vi "autodetector.vi"() -> ()   [LabVIEW 2013]
uses:
  TDMS datalogger/module/configuration/TDMS datalogger configuration.lvclass
  TDMS datalogger/module/execution/TDMS datalogger runtime.lvclass
  configuration/Scan Engine configuration.lvclass
  execution/Scan Engine runtime.lvclass
  <vilib>/NI/Tag Bus Module Framework/channel/TBM channel.lvclass
  <vilib>/NI/Tag Bus/tag/Data Type.ctl
  <vilib>/NI/Tag Bus/tag/tag descriptor.lvclass
  <vilib>/NI/Tag Bus Module Framework/channel/channel classification.ctl
  <vilib>/NI/Tag Bus/table/data table.lvlib
  <vilib>/NI/Tag Bus/table/data polymorphs/write one/write Double.vi
  <vilib>/NI/Tag Bus/dictionary/data dictionary.lvclass
  <vilib>/NI/Module Execution Interface/Engine Configuration/engine configuration.lvclass
  <vilib>/NI/TBM Modules/iov/module/configuration/Scan Engine configuration.lvclass
  <vilib>/NI/Module Execution Interface/Engine Runtime/Engine Runtime Interface.lvclass
  <vilib>/NI/Tag Bus Module Framework/runtime/execution settings.ctl
  <vilib>/NI/Tag Bus Module Framework/runtime/TBM module execution interface.lvclass
panel:
  out "maps dynamically?":bool
  out "error out 2":errorcluster
  out "Array":string[](array[string])
  in  "stop":bool
  out "error out":errorcluster
  out "execution settings":T1
  out "all classes":T2[](array[typedef])
  out "all names":string[](array[string])
  out "remote class":T2[](array[typedef])
  out "remote name":string[](array[string])
  out "local name":string[](array[string])
  out "local class":T2[](array[typedef])
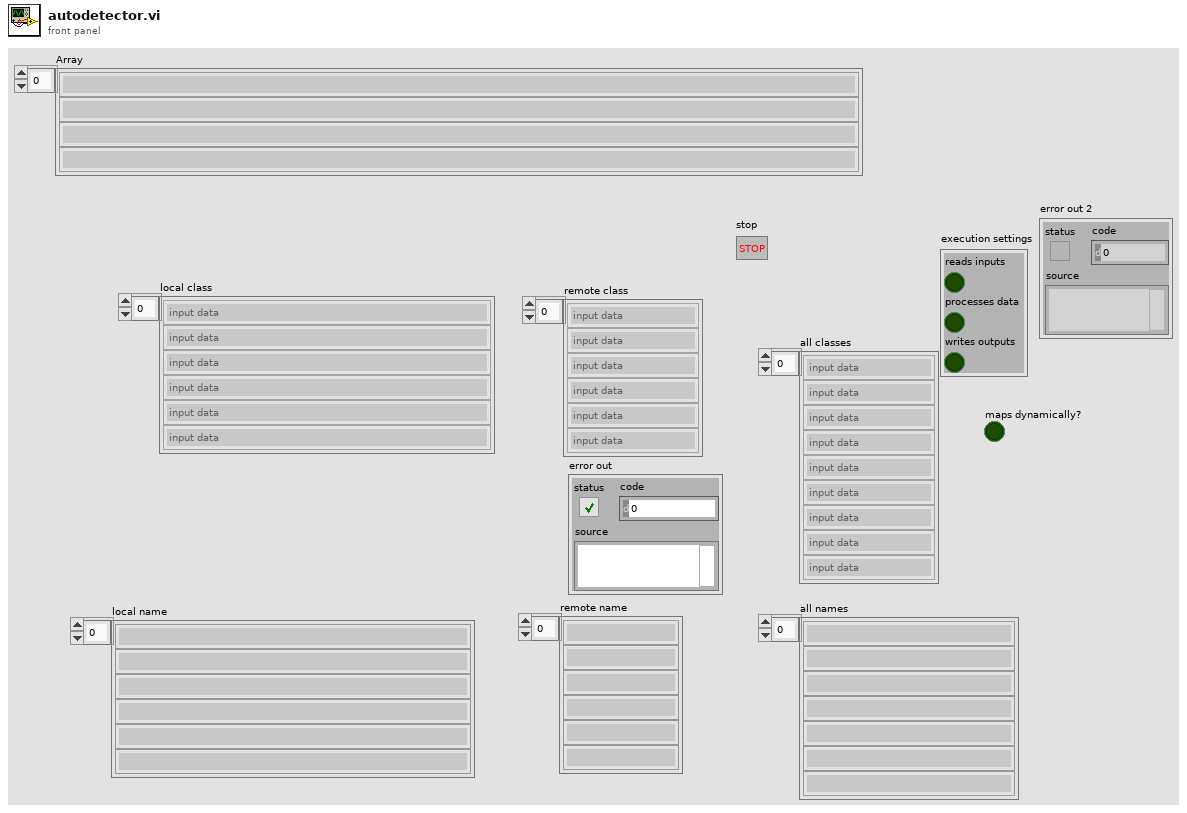
[diagram p1: front panel]
types:
  T1 = typedef "TBM module execution interface.lvclass/execution settings.ctl" = cluster{"reads inputs":bool, "processes data":bool, "writes outputs":bool}
  T2 = typedef "TBM channel.lvclass/channel classification.ctl" = enum16{"input data", "output data", "processing parameter", "processing result"}
  T3 = typedef "tag bus.lvlib/tag descriptor.lvclass/Data Type.ctl" = enum16{"Double", "Single", "I64", "I32", "I16", "I8", "U64", "U32", "U16", "U8", "Boolean", "String", "Array of Double", "Array of Single", "Array of I64", "Array of I32", "Array of I16", "Array of I8", "Array of U64", "Array of U32", "Array of U16", "Array of U8", "Array of Boolean", "Array of String"}
  T4 = typedef "TBM module configuration.lvclass/channel reservation.ctl" = cluster{"local channel":refnum<class "TBM channel.lvclass">, "remote channel":refnum<class "TBM channel.lvclass">}
  T5 = typedef "TBM channel.lvclass/data tables.ctl" = cluster{"input data":T6, "processing parameter":T6, "processing result":T6, "output data":T6}
  T6 = typedef "tag bus.lvlib/dictionary table pair.ctl" = cluster{"data dictionary":refnum<class "data dictionary.lvclass">, "data table":T7}
  T7 = typedef "tag bus.lvlib/data table.lvlib/data table.ctl" = cluster{"Double":dbl[], "Single":sgl[], "I64":i64[], "I32":i32[], "I16":i16[], "I8":i8[], "U64":u64[], "U32":u32[], "U16":u16[], "U8":u8[], "Boolean":bool[], "String":string[], "Array of Double":cluster{"DBL Array":dbl[]}[], "Array of Single":cluster{"SGL Array":sgl[]}[], "Array of I64":cluster{"I64 Array":i64[]}[], "Array of I32":cluster{"I32 Array":i32[]}[], "Array of I16":cluster{"I16 Array":i16[]}[], "Array of I8":cluster{"I8 Array":i8[]}[], "Array of U64":cluster{"U64 Array":u64[]}[], "Array of U32":cluster{"U32 Array":u32[]}[], "Array of U16":cluster{"U16 Array":u16[]}[], "Array of U8":cluster{"U8 Array":u8[]}[], "Array of Boolean":cluster{"Boolean Array":bool[]}[], "Array of String":cluster{"String Array":string[]}[]}
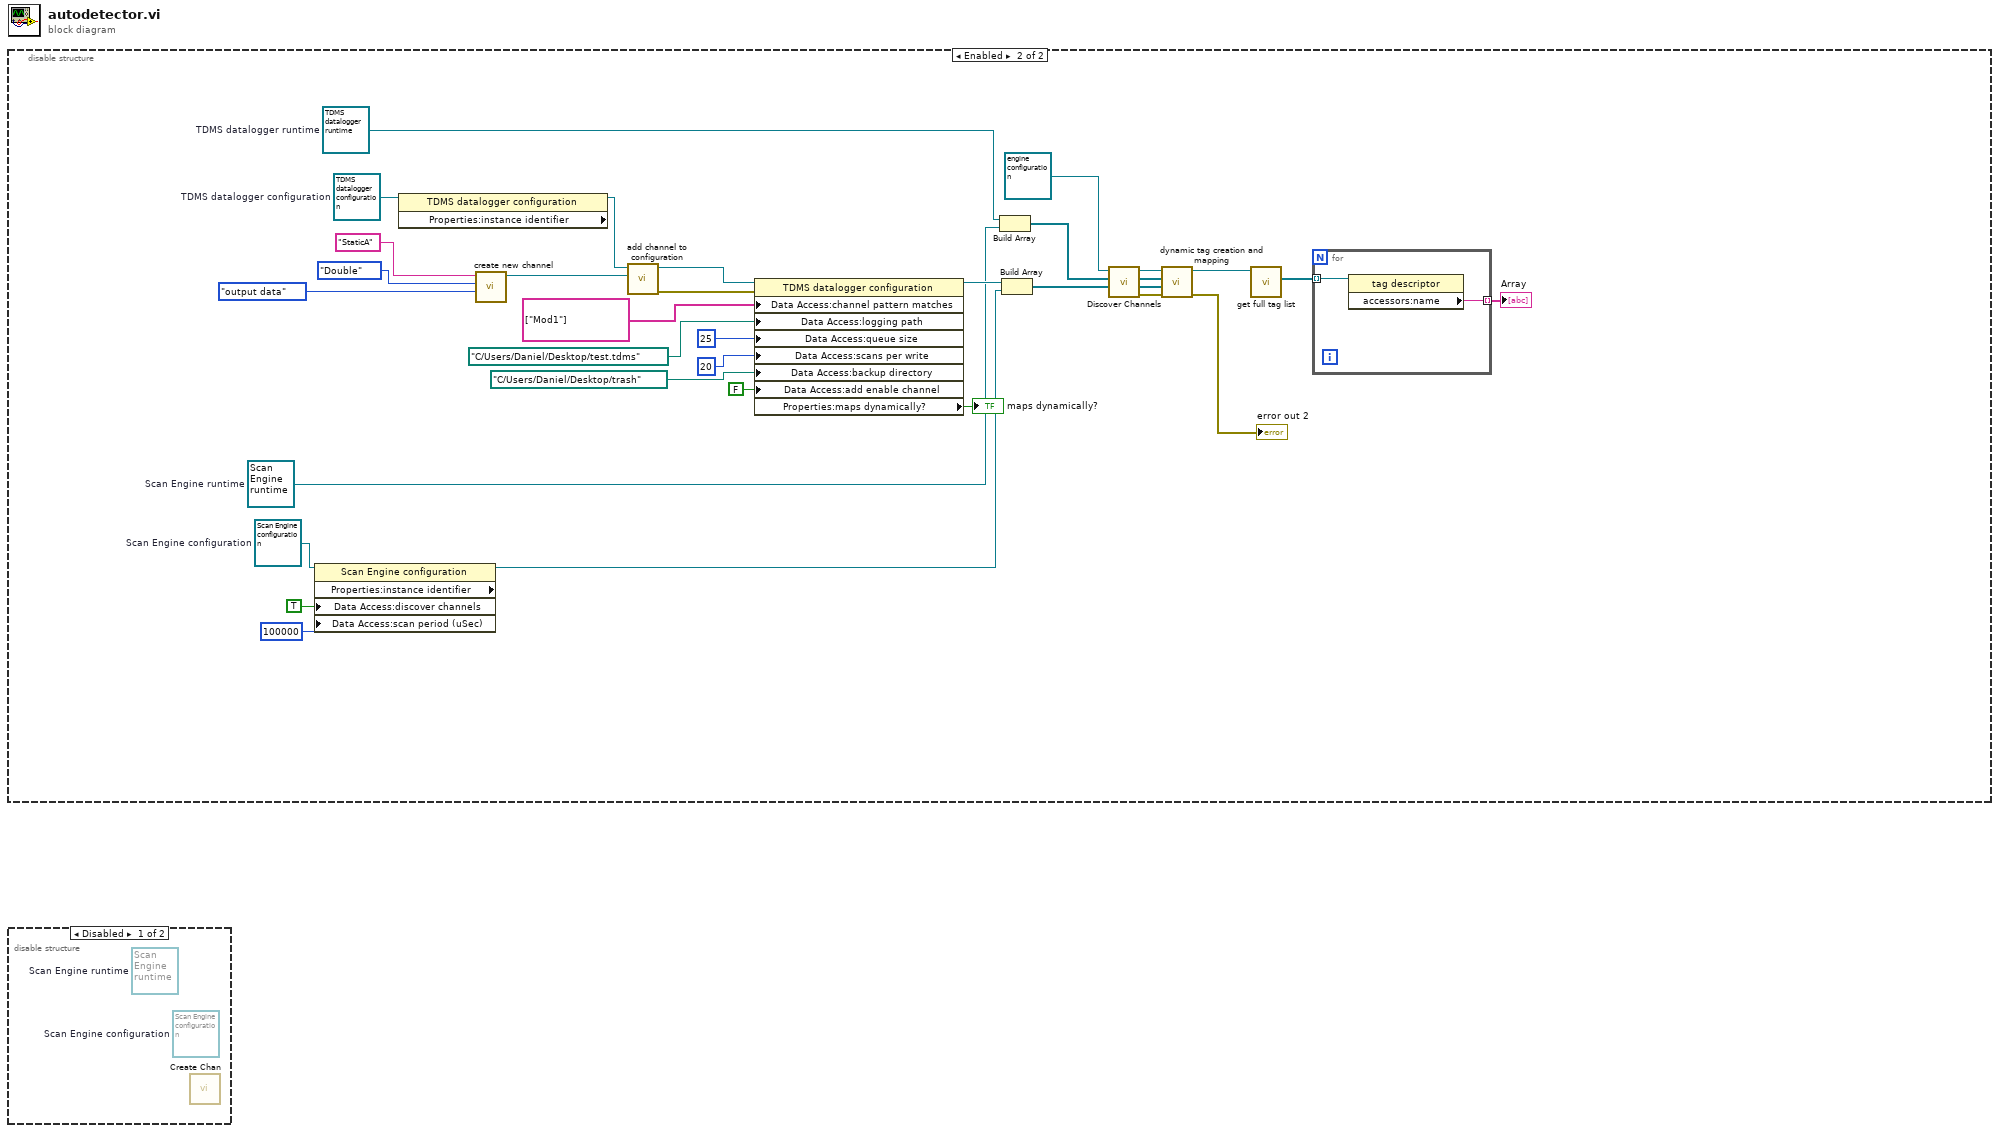
[diagram p0: block diagram]
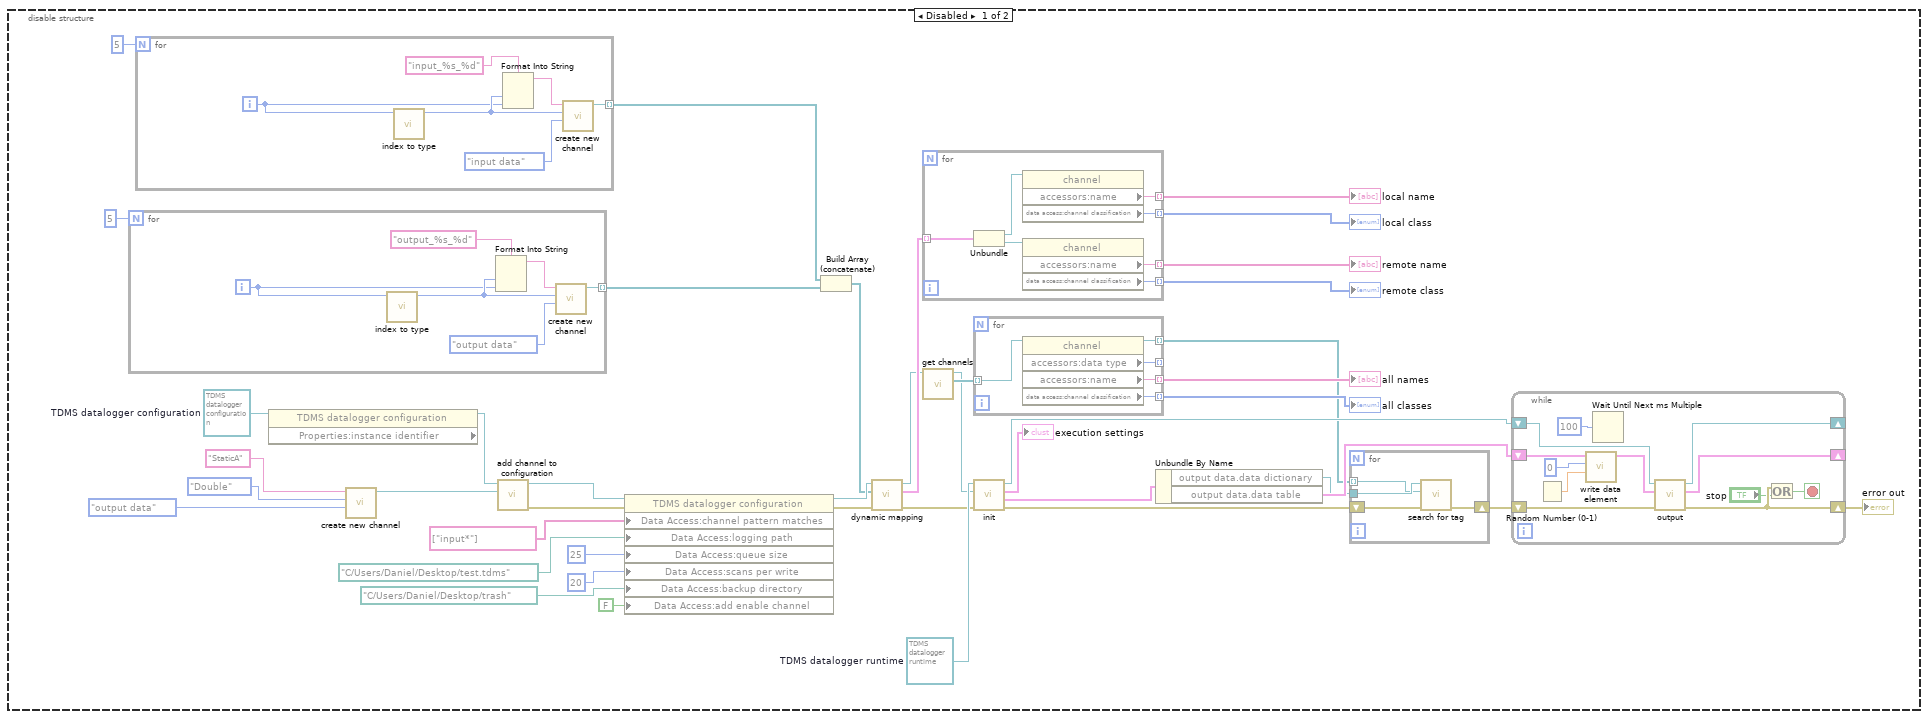
[diagram p2: hidden frame]
diagram:
  n1 = disable-structure shown="Enabled" {
    frame Disabled {
      w17 = refnum<class "TDMS datalogger runtime.lvclass"> refnum  # TDMS datalogger runtime
      w42 = refnum<class "TDMS datalogger configuration.lvclass"> refnum  # TDMS datalogger configuration
      n2 = for {
        N: 5 -> [_]
        tunnel: [w71] -> w35 mode=indexing
        i -> [w73]
        n3 = call <vilib>:"index to type.vi"("I32"=w73) -> ("type"=w75:T3)  [unwired: 10 in]
        n4 = Format Into String(format string="output_%s_%d", w75, w73) -> (resulting string=w72:string)  [unwired: 2 in, 1 out]
        n5 = call <vilib>:"create new channel.vi"("channel classification"=channel_classification."output data", "data type"=w75, "channel name"=w72) -> ("channel"=w71:refnum<class "TBM channel.lvclass">)  [unwired: 8 in]
      }
      n6 = for {
        N: 5 -> [_]
        tunnel: [w77] -> w34 mode=indexing
        i -> [w79]
        n7 = call <vilib>:"index to type.vi"("I32"=w79) -> ("type"=w81:T3)  [unwired: 10 in]
        n8 = Format Into String(format string="input_%s_%d", w81, w79) -> (resulting string=w78:string)  [unwired: 2 in, 1 out]
        n9 = call <vilib>:"create new channel.vi"("channel classification"=channel_classification."input data", "data type"=w81, "channel name"=w78) -> ("channel"=w77:refnum<class "TBM channel.lvclass">)  [unwired: 8 in]
      }
      n10 = property class="TDMS datalogger configuration" props=["Properties:instance identifier"](reference=w42) -> (reference out=w26:refnum<class "TDMS datalogger configuration.lvclass">)  [unwired: 1 in, 2 out]
      n11 = call <vilib>:"create new channel.vi"("channel classification"=channel_classification."output data", "data type"=Data_Type."Double", "channel name"="StaticA") -> ("channel"=w41:refnum<class "TBM channel.lvclass">)  [unwired: 8 in]
      n12 = call "add channel to configuration.vi"("TBM channel in"=w41, "TDMS datalogger configuration in"=w26) -> ("error out"=w33:errorcluster, "TDMS datalogger configuration out"=w31:refnum<class "TDMS datalogger configuration.lvclass">)  [unwired: 8 in]
      n13 = property class="TDMS datalogger configuration"(reference=w31, error in=w33, "Data Access:channel pattern matches"=string[] ["input*"] ("channel pattern matches"), "Data Access:logging path"=path "C:/Users/Daniel/Desktop/test.tdms" ("logging path"), "Data Access:queue size"=25 ("queue size"), "Data Access:scans per write"=20 ("scans per write"), "Data Access:backup directory"=path "C:/Users/Daniel/Desktop/trash" ("backup directory"), "Data Access:add enable channel"=FALSE ("add enable channel")) -> (reference out=w30:refnum<class "TDMS datalogger configuration.lvclass">, error out=w32:errorcluster)
      n14 = Build Array (concatenate)(w34, w35) -> (w28:refnum<class "TBM channel.lvclass">[])
      n15 = call-dynamic "dynamic mapping.vi"("error in"=w32, "channels available"=w28, "module configuration in"=w30) -> ("error out"=w15:errorcluster, "reservations"=w27:T4[], "module configuration out"=w21:refnum<class "TDMS datalogger configuration.lvclass">)  [unwired: 6 in]
      n16 = for {
        tunnel: w27 -> [w70] mode=indexing
        tunnel: [w68] -> w25 mode=indexing
        tunnel: [w67] -> w24 mode=indexing
        tunnel: [w65] -> w23 mode=indexing
        tunnel: [w64] -> w22 mode=indexing
        n17 = Unbundle(w70) -> ("local channel"=w69:refnum<class "TBM channel.lvclass">, "remote channel"=w66:refnum<class "TBM channel.lvclass">)
        n18 = property class="channel"(reference=w69) -> ("accessors:name"=w67:string, "data access:channel classification"=w68:T2)  [unwired: 1 in, 2 out]
        n19 = property class="channel"(reference=w66) -> ("accessors:name"=w65:string, "data access:channel classification"=w64:T2)  [unwired: 1 in, 2 out]
      }
      "local class" <- w25
      "local name" <- w24
      "remote class" <- w22
      "remote name" <- w23
      n20 = call-dynamic "get channels.vi"("module configuration in"=w21) -> ("channels"=w20:refnum<class "TBM channel.lvclass">[], "module configuration out"=w16:refnum<class "TDMS datalogger configuration.lvclass">)  [unwired: 9 in]
      n21 = for {
        tunnel: w20 -> [w63] mode=indexing
        tunnel: [w62] -> w19 mode=indexing
        tunnel: [w61] -> w18 mode=indexing
        tunnel: [w60] -> _ mode=indexing
        tunnel: [w59] -> w8 mode=indexing
        n22 = property class="channel"(reference=w63) -> (reference out=w59:refnum<class "TBM channel.lvclass">, "accessors:data type"=w60:T3, "accessors:name"=w62:string, "data access:channel classification"=w61:T2)  [unwired: 1 in, 1 out]
      }
      "all classes" <- w18
      "all names" <- w19
      n23 = call-dynamic "init.vi"("error in"=w15, "TBM module configuration in"=w16, "TDMS datalogger runtime in"=w17) -> ("error out"=w7:errorcluster, "data allocations"=w13:T5, "execution settings"=→"execution settings":T1, "TDMS datalogger runtime out"=w11:refnum<class "TDMS datalogger runtime.lvclass">)  [unwired: 5 in]
      n24 = Unbundle By Name(w13) -> ("output data.data dictionary"=w9:refnum<class "data dictionary.lvclass">, "output data.data table"=w12:T7)
      n25 = for {
        tunnel: w9 -> [w46]
        tunnel: w8 -> [w45] mode=indexing
        shift-right: [w44] -> w6
        shift-left: w7 -> [w43]
        n26 = call <vilib>:"search for tag.vi"("error in"=w43, "system tag"=w45, "data dictionary in"=w46) -> ("error out"=w44:errorcluster)  [unwired: 6 in, 2 out]
      }
      n27 = while {
        shift-right: [w53] -> _
        shift-left: w11 -> [w56]
        shift-right: [w52] -> _
        shift-left: w12 -> [w58]
        shift-right: [w50] -> w10
        shift-left: w6 -> [w49]
        stop <- w48 stop-if-true
        n28 = Random Number (0-1)() -> (number: 0 to 1=w55:dbl)
        n29 = call-poly <vilib>:"write data element.vi"("value"=w55, "index"=0, "data table in"=w58) -> ("data table out"=w51:T7)  [unwired: 8 in]
        n30 = Wait Until Next ms Multiple(millisecond multiple=u32 100) -> ()  [unwired: 1 out]
        n31 = call-dynamic "output.vi"("error in"=w49, "data table in"=w51, "TDMS datalogger runtime in"=w56) -> ("error out"=w50:errorcluster, "data table out"=w52:T7, "TDMS datalogger runtime out"=w53:refnum<class "TDMS datalogger runtime.lvclass">)  [unwired: 6 in]
        n32 = Or(x=w50, y="stop") -> (x .or. y?=w48:bool)
      }
      "error out" <- w10
    }
    frame Enabled {
      w98 = refnum<class "TDMS datalogger runtime.lvclass"> refnum  # TDMS datalogger runtime
      w100 = refnum<class "Scan Engine configuration.lvclass"> refnum  # Scan Engine configuration
      w97 = refnum<class "Scan Engine runtime.lvclass"> refnum  # Scan Engine runtime
      w115 = refnum<class "TDMS datalogger configuration.lvclass"> refnum  # TDMS datalogger configuration
      n33 = property class="Scan Engine configuration" props=["Properties:instance identifier", "Data Access:discover channels", "Data Access:scan period (uSec)"](reference=w100, "Data Access:discover channels"=TRUE ("discover channels"), "Data Access:scan period (uSec)"=u32 100000 ("scan period (uSec)")) -> (reference out=w96:refnum<class "Scan Engine configuration.lvclass">)  [unwired: 1 in, 2 out]
      n34 = property class="TDMS datalogger configuration" props=["Properties:instance identifier"](reference=w115) -> (reference out=w107:refnum<class "TDMS datalogger configuration.lvclass">)  [unwired: 1 in, 2 out]
      n35 = call <vilib>:"create new channel.vi"("channel classification"=channel_classification."output data", "data type"=Data_Type."Double", "channel name"="StaticA") -> ("channel"=w114:refnum<class "TBM channel.lvclass">)  [unwired: 8 in]
      n36 = call "add channel to configuration.vi"("TBM channel in"=w114, "TDMS datalogger configuration in"=w107) -> ("error out"=w110:errorcluster, "TDMS datalogger configuration out"=w109:refnum<class "TDMS datalogger configuration.lvclass">)  [unwired: 8 in]
      n37 = property class="TDMS datalogger configuration"(reference=w109, error in=w110, "Data Access:channel pattern matches"=string[] ["Mod1"] ("channel pattern matches"), "Data Access:logging path"=path "C:/Users/Daniel/Desktop/test.tdms" ("logging path"), "Data Access:queue size"=25 ("queue size"), "Data Access:scans per write"=20 ("scans per write"), "Data Access:backup directory"=path "C:/Users/Daniel/Desktop/trash" ("backup directory"), "Data Access:add enable channel"=FALSE ("add enable channel")) -> (reference out=w101:refnum<class "TDMS datalogger configuration.lvclass">, "Properties:maps dynamically?"=→"maps dynamically?":bool)  [unwired: 1 out]
      n38 = Build Array(w98, w97) -> (w87:refnum<class "TBM module execution interface.lvclass">[])
      n39 = Build Array(w101, w96) -> (w86:refnum<class "TBM module configuration.lvclass">[])
      n40 = call <vilib>:"Discover Channels.vi"("module configurations"=w86, "modules"=w87, "engine configuration"=refnum<class "engine configuration.lvclass"> refnum ("engine configuration in")) -> ("error out"=w89:errorcluster, "module configurations out"=w83:refnum<class "TBM module configuration.lvclass">[], "modules out"=w84:refnum<class "TBM module execution interface.lvclass">[], "engine configuration out"=w90:refnum<class "engine configuration.lvclass">)  [unwired: 5 in]
      n41 = call <vilib>:"dynamic tag creation and mapping.vi"("error in (no error)"=w89, "module configurations"=w83, "modules"=w84, "engine configuration in"=w90) -> ("error out"=→"error out 2":errorcluster, "engine configuration out"=w85:refnum<class "engine configuration.lvclass">)  [unwired: 4 in, 2 out]
      n42 = call <vilib>:"get full tag list.vi"("engine configuration in"=w85) -> ("tag list"=w95:refnum<class "tag descriptor.lvclass">[])  [unwired: 9 in, 1 out]
      n43 = for {
        tunnel: w95 -> [w117] mode=indexing
        tunnel: [w116] -> w94 mode=indexing
        n44 = property class="tag descriptor"(reference=w117) -> ("accessors:name"=w116:string)  [unwired: 1 in, 2 out]
      }
      "Array" <- w94
    }
  }
  n45 = disable-structure shown="Disabled" {
    frame Disabled {
      (unwired) refnum<class "Scan Engine runtime.lvclass"> refnum  # Scan Engine runtime
      (unwired) refnum<class "Scan Engine configuration.lvclass"> refnum  # Scan Engine configuration
      n46 = call <vilib>:"Create Chan.vi"() -> ()  [unwired: 10 in, 2 out]
    }
    frame Enabled {
    }
  }
